vi "Panel.vi"(10 "Actor":refnum<class "Actor.lvclass">, 11 "Panel":refnum<class "Panel.lvclass">) -> ()   [LabVIEW 2021, in "Panel.lvclass"]
uses:
  Panel.lvclass
  <vilib>/jettl/jettl/Actor/Actor/Actor.lvclass
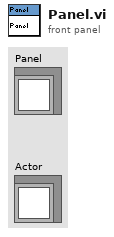
[diagram p1: front panel]
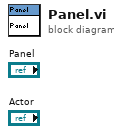
[diagram p0: block diagram]
diagram:
